vi "SendCmd.vi"(8 "error in (no error)":errorcluster, 10 "index":i32, 11 "DataIn":string) -> (0 "error out":errorcluster, 2 "TimeOut":bool, 3 "Reccmd":string)   [LabVIEW 2019]
panel:
  out "OffReply":string
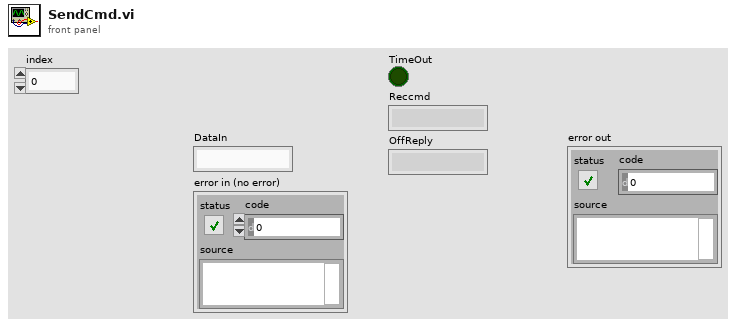
[diagram p1: front panel]
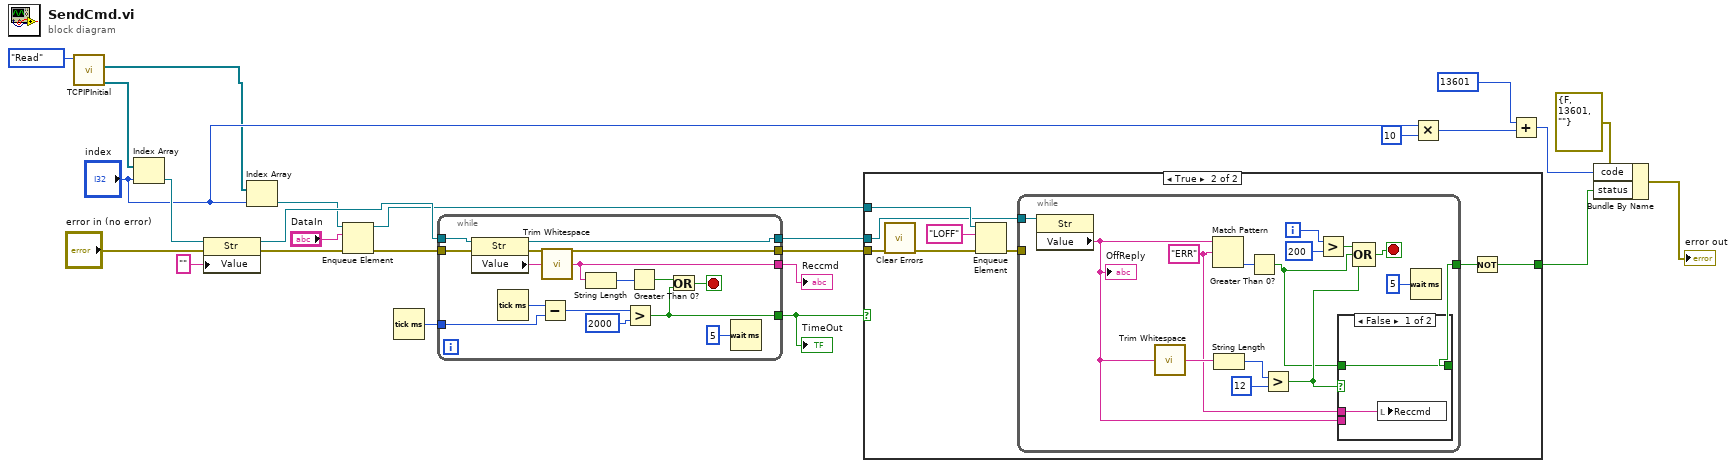
[diagram p0: block diagram]
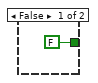
[diagram p2: hidden frame]
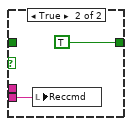
[diagram p3: hidden frame]
diagram:
  n1 = call "TCPIPInitial.vi"("Enum"=enum16{"initial", "Read", "release"}."Read") -> ("SN_ReplyRef"=w1:refnum<vi>[], "Sn_cmdQ"=w2:refnum<queue>[])  [unwired: 7 in, 2 out]
  n2 = Index Array(array=w1, index="index") -> (element=w13:refnum<vi>)
  n3 = property class="Str"(reference=w13, error in="error in (no error)", "Value"="") -> (reference out=w21:refnum<vi>, error out=w23:errorcluster)
  n4 = Index Array(array=w2, index="index") -> (element=w12:refnum<queue>)
  n5 = Enqueue Element(queue=w12, element="DataIn", error in (no error)=w23) -> (queue out=w18:refnum<queue>, error out=w19:errorcluster)  [unwired: 1 in, 1 out]
  n6 = Tick Count (ms)() -> (millisecond timer value=w20:u32)
  n7 = while {
    tunnel: w21 -> [w39]
    tunnel: w20 -> [w37]
    tunnel: w19 -> [w31]
    tunnel: [w30] -> w17
    tunnel: [w29] -> w14
    tunnel: [w28] -> w16
    tunnel: [w26] -> w15
    stop <- w32 stop-if-true
    n8 = property class="Str"(reference=w39, error in=w31) -> (reference out=w26:refnum<vi>, error out=w30:errorcluster, "Value"=w40:string)
    n9 = Tick Count (ms)() -> (millisecond timer value=w36:u32)
    n10 = Subtract(x=w36, y=w37) -> (x-y=w35:u32)
    n11 = call <vilib>:"Trim Whitespace.vi"("string"=w40) -> ("trimmed string"=w28:string)  [unwired: 1 in]
    n12 = String Length(string=w28) -> (length=w38:i32)
    n13 = Greater?(x=w35, y=u32 2000) -> (0:w29:bool)
    n14 = Greater Than 0?(x=w38) -> (x > 0?=w33:bool)
    n15 = Or(x=w33, y=w29) -> (x .or. y?=w32:bool)
    n16 = Wait (ms)(milliseconds to wait=u32 5 ("millisecond timer value")) -> ()  [unwired: 1 out]
  }
  "TimeOut" <- w14
  "Reccmd" <- w16
  n17 = case shown="True" w14 {
    tunnel: w18 -> [_ w49]
    tunnel: w17 -> [_ w47]
    tunnel: w15 -> [_ w45]
    tunnel: [FALSE w42] -> w9
    frame False {
    }
    frame True {
      n18 = call <vilib>:"Clear Errors.vi"("error in (no error)"=w47) -> ("error out"=w46:errorcluster)  [unwired: 5 in, 1 out]
      n19 = Enqueue Element(queue=w49, element="LOFF", error in (no error)=w46) -> (error out=w44:errorcluster)  [unwired: 1 in, 2 out]
      n20 = while {
        tunnel: w45 -> [w64]
        tunnel: w44 -> [_]
        tunnel: [w54] -> w43
        i -> [w62]
        stop <- w58 stop-if-true
        w50 = "ERR" ("regular expression")
        n21 = property class="Str"(reference=w64) -> ("Value"=w56:string)  [unwired: 1 in, 2 out]
        "OffReply" <- w56
        n22 = call <vilib>:"Trim Whitespace.vi"("string"=w56) -> ("trimmed string"=w57:string)  [unwired: 1 in]
        n23 = Match Pattern(string=w56, regular expression=w50) -> (offset past match=w59:i32)  [unwired: 1 in, 3 out]
        n24 = String Length(string=w57) -> (length=w52:i32)
        n25 = Greater Than 0?(x=w59) -> (x > 0?=w53:bool)
        n26 = Greater?(x=w52, y=12) -> (0:w55:bool)
        n27 = Greater?(x=w62, y=200) -> (0:w60:bool)
        n28 = case shown="False" w55 {
          tunnel: w56 -> [_ w68]
          tunnel: [w66 TRUE] -> w54
          tunnel: w53 -> [w66 _]
          tunnel: w50 -> [w65 _]
          frame False {
            n29 = local write "Reccmd"(w65) -> ()
          }
          frame True {
            n30 = local write "Reccmd"(w68) -> ()
          }
        }
        n31 = Compound Arithmetic op=OR(w60, w53, w55) -> (w58:bool)
        n32 = Wait (ms)(milliseconds to wait=u32 5 ("millisecond timer value")) -> ()  [unwired: 1 out]
      }
      n33 = Not(x=w43) -> (.not. x?=w42:bool)
    }
  }
  n34 = Multiply(x="index", y=10) -> (x*y=w4:i32)
  n35 = Add(x=13601 ("code"), y=w4) -> (x+y=w8:i32)
  n36 = Bundle By Name(cluster=errorcluster {"status"=FALSE, "code"=13601, "source"=""} ("error constant"), "code"=w8, "status"=w9) -> (→"error out":errorcluster)
